vi "Read Controller Name.vi"(11 "Timed Loop Controller":refnum<class "Timed Loop Actor.lvclass">) -> (2 "Controller Name":string)   [LabVIEW 2018, in "Timed Loop Actor.lvlib" / "Timed Loop Actor.lvclass"]
doc: "This reads the controller name. This name is used just for debugging purposes except on real-time systems, where it is part of the framework for stopping the Timed Loop."
uses:
  Timed Loop Actor.lvclass
  Timed Loop Actor.lvclass/Timed Loop Actor.ctl
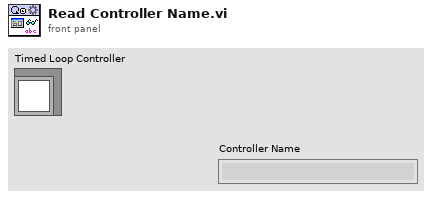
[diagram p1: front panel]
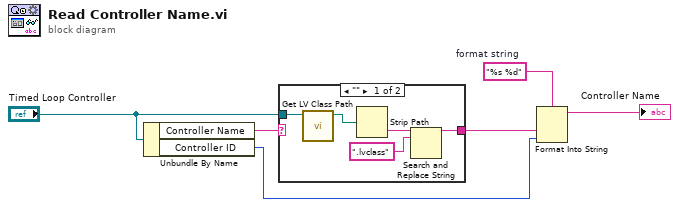
[diagram p0: block diagram]
diagram:
  w6 = "%s %d"  # format string
  n1 = Unbundle By Name("Timed Loop Controller") -> ("Controller Name"=w2:string, "Controller ID"=w5:u32)
  n2 = case shown="\"\"" w2 {
    selector: w2 -> [_ w12]
    tunnel: "Timed Loop Controller" -> [w11 _]
    tunnel: [w8 w12] -> w1
    frame "" {
      n3 = call <vilib>:"Get LV Class Path.vi"("object"=w11) -> ("class path"=w10:path)  [unwired: 9 in, 1 out]
      n4 = Strip Path(path=w10) -> (name=w9:string)  [unwired: 1 out]
      n5 = Search and Replace String(input string=w9, search string=".lvclass") -> (result string=w8:string)  [unwired: 6 in, 3 out]
    }
    frame Default {
    }
  }
  n6 = Format Into String(format string=w6, w1, w5) -> (resulting string=→"Controller Name":string)  [unwired: 2 in, 1 out]
